vi "fgv_system_state.vi"(7 "cmd":enum16{"init", "read", "write"}(ring), 8 "error in":errorcluster, 11 "State":T1) -> (0 "error out":errorcluster, 3 "State out":T1)   [LabVIEW 2019]
uses:
  Ctrl/state.ctl
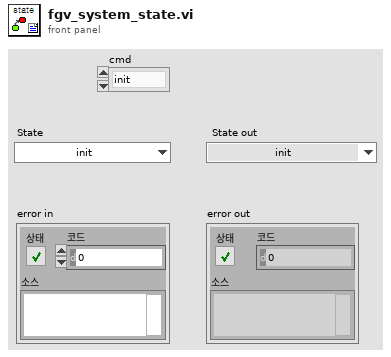
[diagram p1: front panel]
types:
  T1 = typedef "state.ctl" = enum16{"init", "Test circular track", "start point", "start heading adjust", "wait before start", "stop point check", "stop point start", "end point", "entering ending point", "move", "move heading adjust"}
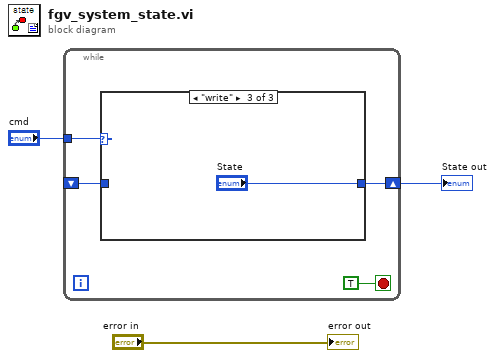
[diagram p0: block diagram]
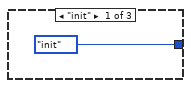
[diagram p2: hidden frame]
diagram:
  n1 = while {
    tunnel: "cmd" -> [w6]
    shift-right: [w5] -> w2
    shift-left: _ -> [w4]
    stop <- TRUE stop-if-true
    n2 = case shown="\"write\"" w6 {
      tunnel: [state."init" ("State") w9 "State"] -> w5
      tunnel: w4 -> [_ w9 _]
      frame "init" {
      }
      frame "read", Default {
      }
      frame "write" {
      }
    }
  }
  "State out" <- w2
  "error out" <- "error in"
